vi "Display Result.vi"(8 "error in (no error)":errorcluster, 10 "Stack":dbl[](array[numeric]), 11 "Calculator in":refnum<class "Calculator.lvclass">) -> (0 "error out":errorcluster, 3 "Calculator out":refnum<class "Calculator.lvclass">)   [LabVIEW 2012, in "Calculator.lvlib" / "Calculator.lvclass"]
doc: "Set value on Frontpanel via reference."
uses:
  Calculator.lvclass
  Calculator.lvclass/Calculator.ctl
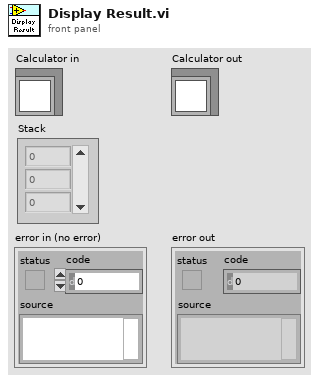
[diagram p1: front panel]
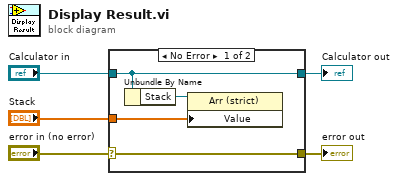
[diagram p0: block diagram]
diagram:
  n1 = case shown="No Error" "error in (no error)" {
    selector: "error in (no error)" -> [w9 w11]
    tunnel: [w9 w11] -> w4
    tunnel: [w8 w10] -> w2
    tunnel: "Calculator in" -> [w8 w10]
    tunnel: "Stack" -> [w6 _]
    frame No Error {
      n2 = Unbundle By Name(w8) -> ("Stack"=w7:refnum<vi>)
      n3 = property class="Arr (strict)"(reference=w7, "Value"=w6) -> ()  [unwired: 1 in, 2 out]
    }
    frame Error {
    }
  }
  "error out" <- w4
  "Calculator out" <- w2
